vi "Create_Default_RegDests.vi"(8 "error in (no error)":errorcluster, 11 "IB_MSI in":refnum<class "IB_MSI.lvclass">) -> (0 "error out":errorcluster, 3 "IB_MSI out":refnum<class "IB_MSI.lvclass">)   [LabVIEW 2020, in "IB_MSI.lvclass"]
uses:
  <vilib>/AppBuilder/IB_Classes/MSI/IB_MSI.lvclass
  <vilib>/AppBuilder/IB_Classes/MSI/IB_MSI.lvclass/IB_MSI.ctl
  <vilib>/AppBuilder/IB_Classes/RegDest/RegDest_Label/IB_RegDest_Label.lvclass
  <vilib>/AppBuilder/IB_Classes/RegDest/RegDest_User/IB_RegDest_User.lvclass
  <vilib>/AppBuilder/IB_Classes/RegDest/IB_RegDest.lvclass
  <resource>/Framework/Providers/Builds/Installer/CDK_sTypeDef_DirInfo.ctl
  e:/builds/penguin/labview/branches/2020/dev/dist/vi.lib/AppBuilder/IB_Classes/RegDest/IB_RegDest.lvclass
  e:/builds/penguin/labview/branches/2020/dev/dist/vi.lib/AppBuilder/IB_Classes/RegDest/RegDest_Label/IB_RegDest_Label.lvclass
  e:/builds/penguin/labview/branches/2020/dev/dist/vi.lib/AppBuilder/IB_Classes/RegDest/RegDest_User/IB_RegDest_User.lvclass
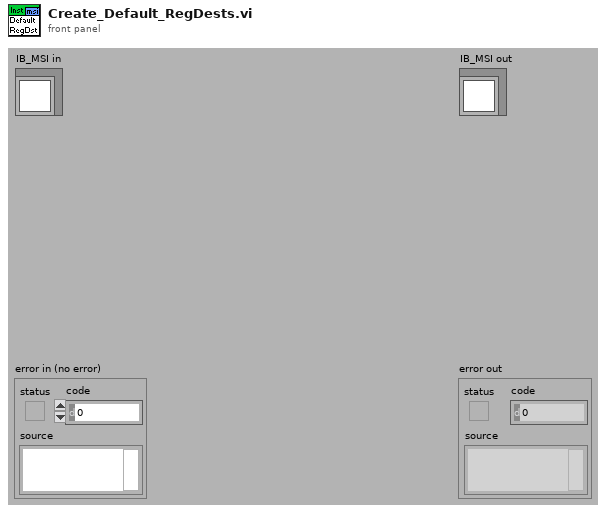
[diagram p1: front panel]
types:
  T1 = typedef "CDK_sTypeDef_DirInfo.ctl" = cluster{"ParentTag":string, "DirTag":string, "DirName":string, "Editable?":bool}
  T2 = typedef "IB_RegDest.ctl" = cluster{"parentTag":string, "dirTag":string, "dirName":string, "unlock":bool, "path":string, "regData":refnum<class "IB_RegData.lvclass">[]}
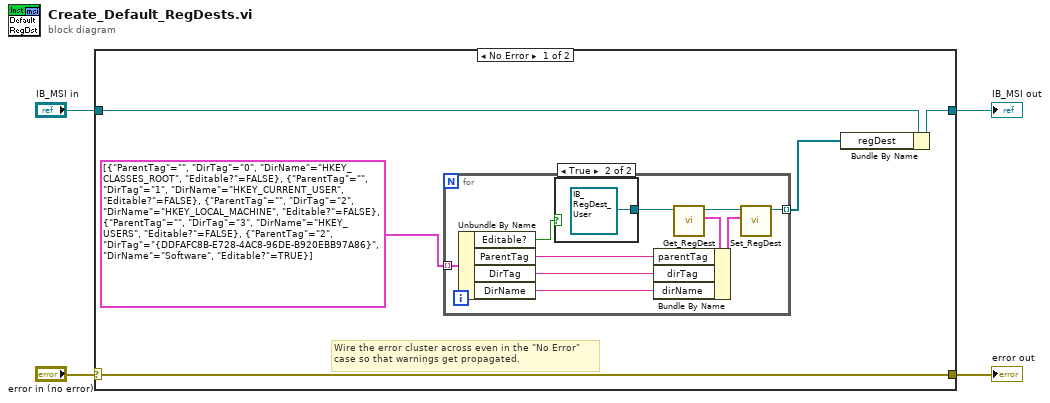
[diagram p0: block diagram]
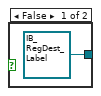
[diagram p2: hidden frame]
diagram:
  n1 = case shown="No Error" "error in (no error)" {
    selector: "error in (no error)" -> [w9 w23]
    tunnel: [w9 w23] -> w3
    tunnel: [w6 w22] -> w1
    tunnel: "IB_MSI in" -> [w7 w22]
    frame No Error {
      # "Wire the error cluster across even in the \"No Error\"\ncase so that warnings get propagated."
      n2 = for {
        tunnel: T1[] [{"ParentTag"="", "DirTag"="0", "DirName"="HKEY_CLASSES_ROOT", "Editable?"=FALSE}, {"ParentTag"="", "DirTag"="1", "DirName"="HKEY_CURRENT_USER", "Editable?"=FALSE}, {"ParentTag"="", "DirTag"="2", "DirName"="HKEY_LOCAL_MACHINE", "Editable?"=FALSE}, {"ParentTag"="", "DirTag"="3", "DirName"="HKEY_USERS", "Editable?"=FALSE}, {"ParentTag"="2", "DirTag"="{DDFAFC8B-E728-4AC8-96DE-B920EBB97A86}", "DirName"="Software", "Editable?"=TRUE}] ("Array") -> [w19] mode=indexing
        tunnel: [w11] -> w5 mode=indexing
        n3 = Unbundle By Name(w19) -> ("Editable?"=w10:bool, "ParentTag"=w14:string, "DirTag"=w13:string, "DirName"=w12:string)
        n4 = case shown="True" w10 {
          tunnel: [refnum<class "IB_RegDest_Label.lvclass"> refnum ("IB_RegDest_Label.lvclass") refnum<class "IB_RegDest_User.lvclass"> refnum ("IB_RegDest_User.lvclass")] -> w17
          frame False {
          }
          frame True {
          }
        }
        n5 = call <vilib>:"Get_RegDest.vi"("Class in"=w17) -> ("data"=w16:T2, "Class out"=w18:refnum<class "IB_RegDest.lvclass">)  [unwired: 1 in, 8 out]
        n6 = Bundle By Name(cluster=w16, "parentTag"=w14, "dirTag"=w13, "dirName"=w12) -> (w15:T2)
        n7 = call <vilib>:"Set_RegDest.vi"("data"=w15, "Class in"=w18) -> ("Class out"=w11:refnum<class "IB_RegDest.lvclass">)  [unwired: 1 in, 8 out]
      }
      n8 = Bundle By Name(cluster=w7, "regDest"=w5) -> (w6:refnum<class "IB_MSI.lvclass">)
    }
    frame Error {
    }
  }
  "error out" <- w3
  "IB_MSI out" <- w1
